vi "rec_time.vi"() -> ()   [LabVIEW 2017]
panel:
  out "output array":dbl[](array[numeric])
  out "time":dbl
  in  "duty rate":dbl
  out "Switch":string="A"
  in  "stop":bool
  in  "Boolean":bool
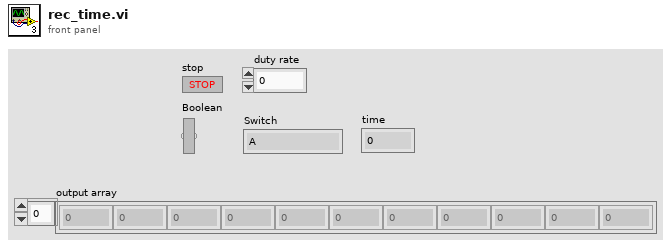
[diagram p1: front panel]
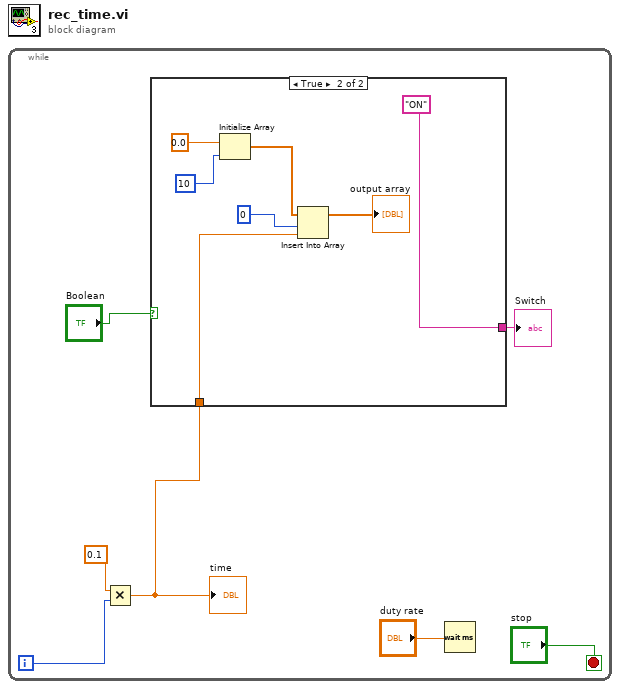
[diagram p0: block diagram]
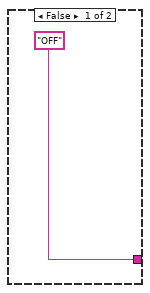
[diagram p2: hidden frame]
diagram:
  n1 = while {
    i -> [w2]
    stop <- "stop" stop-if-true
    n2 = Multiply(x=0.1, y=w2) -> (x*y=w1:dbl)
    "time" <- w1
    n3 = case shown="True" "Boolean" {
      tunnel: ["OFF" "ON"] -> w6
      tunnel: w1 -> [_ w14]
      frame False {
      }
      frame True {
        n4 = Initialize Array(0.0, 10) -> (w11:dbl[])
        n5 = Insert Into Array(array=w11, index=0, new element=w14) -> (→"output array":dbl[])
      }
    }
    "Switch" <- w6
    n6 = Wait (ms)(milliseconds to wait="duty rate") -> ()  [unwired: 1 out]
  }
